vi "Library_SpaceMouse_init.vi"(8 "error in (no error)":errorcluster) -> (0 "error out":errorcluster)   [LabVIEW 2013]
uses:
  My Computer/Controls/SpaceMouse_RawInput.ctl
  My Computer/Controls/SpaceMouse_Parameters.ctl
  My Computer/Controls/SpaceMouse_FilteredInput.ctl
  My Computer/Controls/SpaceMouse_Buttons.ctl
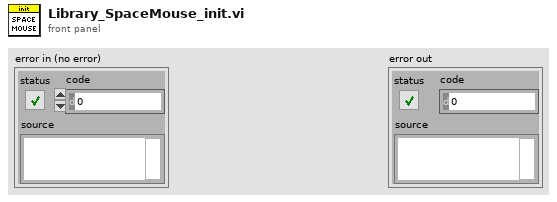
[diagram p1: front panel]
types:
  T1 = typedef "SpaceMouse_Buttons.ctl" = cluster{"Idle":bool, "Button Right":bool, "Button Left":bool}
  T2 = typedef "SpaceMouse_FilteredInput.ctl" = cluster{"X":dbl, "Y":dbl, "Z":dbl, "phi":dbl, "theta":dbl, "psi":dbl}
  T3 = typedef "SpaceMouse_Parameters.ctl" = cluster{"Lowpass Filter Cutoff Frequency":dbl, "Idle Threshold":dbl, "Deadzone":dbl, "Filter Sample Size":i32, "FilterOff":bool, "IntegratorOff":bool}
  T4 = typedef "SpaceMouse_RawInput.ctl" = cluster{"X":i32, "Y":i32, "Z":i32, "phi":i32, "theta":i32, "psi":i32}
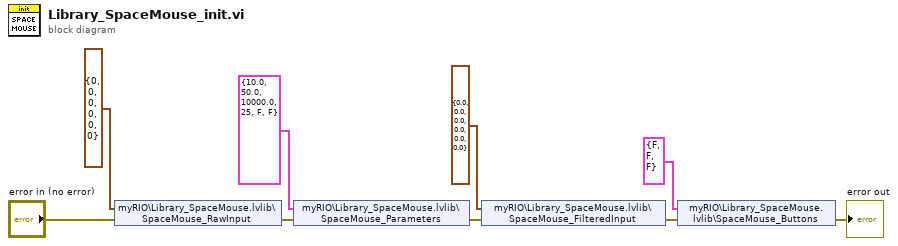
[diagram p0: block diagram]
diagram:
  n1 = shared-variable "myRIO\\Library_SpaceMouse.lvlib\\SpaceMouse_RawInput"(T4 {"X"=0, "Y"=0, "Z"=0, "phi"=0, "theta"=0, "psi"=0} ("SpaceMouse_RawInput"), error in="error in (no error)") -> (error out=w5:errorcluster)
  n2 = shared-variable "myRIO\\Library_SpaceMouse.lvlib\\SpaceMouse_Parameters"(T3 {"Lowpass Filter Cutoff Frequency"=10.0, "Idle Threshold"=50.0, "Deadzone"=10000.0, "Filter Sample Size"=25, "FilterOff"=FALSE, "IntegratorOff"=FALSE} ("SpaceMouse_Parameters"), error in=w5) -> (error out=w4:errorcluster)
  n3 = shared-variable "myRIO\\Library_SpaceMouse.lvlib\\SpaceMouse_FilteredInput"(T2 {"X"=0.0, "Y"=0.0, "Z"=0.0, "phi"=0.0, "theta"=0.0, "psi"=0.0} ("SpaceMouse_FilteredInput"), error in=w4) -> (error out=w3:errorcluster)
  n4 = shared-variable "myRIO\\Library_SpaceMouse.lvlib\\SpaceMouse_Buttons"(T1 {"Idle"=FALSE, "Button Right"=FALSE, "Button Left"=FALSE} ("SpaceMouse_Buttons"), error in=w3) -> (error out=→"error out":errorcluster)
